vi "Initialise.vi"(8 "error in (no error)":errorcluster, 9 "Buffer Size":i32=10, 11 "Image Acquisition in":refnum<class "HAMAMATSU_DCAMAPI.lvclass">) -> (0 "error out":errorcluster, 3 "Image Acquisition out":refnum<class "HAMAMATSU_DCAMAPI.lvclass">)   [LabVIEW 2020, in "HAMAMATSU_DCAMAPI.lvclass"]
uses:
  HAMAMATSU_DCAMAPI.lvclass
  HAMAMATSU_DCAMAPI.lvclass/HAMAMATSU_DCAMAPI.ctl
panel:
  out "DCAM Version":string
  out "Library Version":string
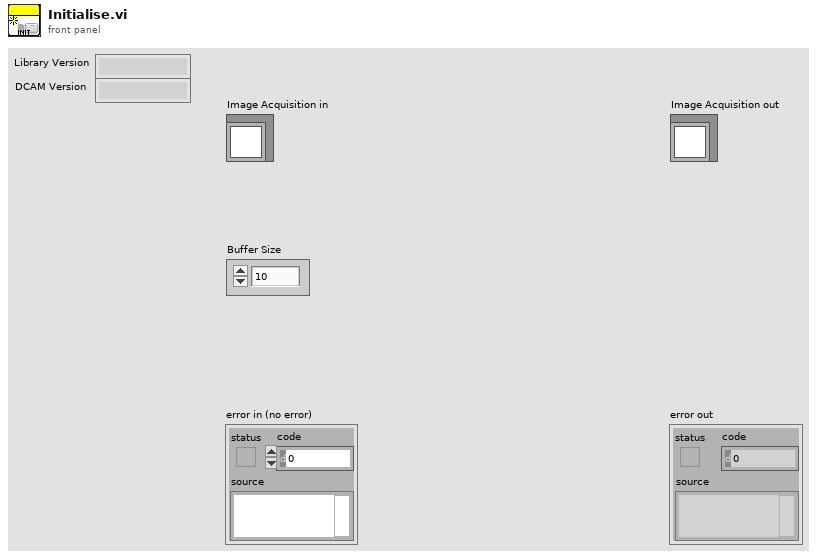
[diagram p1: front panel]
types:
  T1 = cluster{"Capture Library":string, "DCAM-API":string}
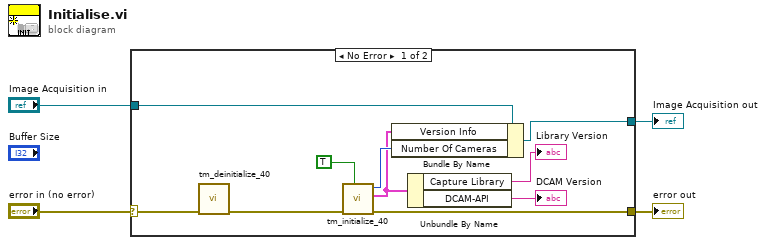
[diagram p0: block diagram]
diagram:
  n1 = case shown="No Error" "error in (no error)" {
    selector: "error in (no error)" -> [w11 w15]
    tunnel: [w10 w15] -> w3
    tunnel: "Image Acquisition in" -> [w9 w16]
    tunnel: [w5 w16] -> w1
    frame No Error {
      n2 = call <userlib>:"tm_deinitialize_40.vi"("error in (no error)"=w11) -> ("error out"=w14:errorcluster)  [unwired: 10 in]
      n3 = call <userlib>:"tm_initialize_40.vi"("HVCC Log (F)"=TRUE, "error in (no error)"=w14) -> ("error out"=w10:errorcluster, "Version Info"=w6:T1, "Number Of Cameras"=w7:u32)  [unwired: 6 in, 1 out]
      n4 = Bundle By Name(cluster=w9, "Version Info"=w6, "Number Of Cameras"=w7) -> (w5:refnum<class "HAMAMATSU_DCAMAPI.lvclass">)
      n5 = Unbundle By Name(w6) -> ("Capture Library"=→"Library Version":string, "DCAM-API"=→"DCAM Version":string)
    }
    frame Error {
    }
  }
  "error out" <- w3
  "Image Acquisition out" <- w1
